vi "SMU.Keithley2600.GetResource.vi"(8 "error in (no error)":errorcluster, 11 "SMU.Keithley2600 in":refnum<class "SMU.Keithley2600.lvclass">) -> (0 "error out":errorcluster, 2 "Resource":T1 {"Channel" items=["Channel A", "Channel B"]}, 3 "SMU.Keithley2600 out":refnum<class "SMU.Keithley2600.lvclass">)   [LabVIEW 2017, in "SMU.Keithley2600.lvclass"]
uses:
  SMU.Keithley2600.lvclass
  Typedefs/Resource--Cluster.ctl
  SMU.Keithley2600.lvclass/SMU.Keithley2600.ctl
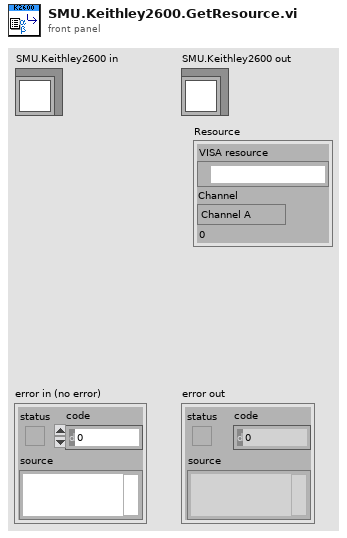
[diagram p1: front panel]
types:
  T1 = typedef "SMU.Keithley2600.lvclass/Resource--Cluster.ctl" = cluster{"VISA resource":refnum<visa-resource-name>, "Channel":i32}
  T2 = typedef "SMU.Keithley2600.lvclass/PrivateData--Ref.ctl" = refnum<data-value>
  T3 = typedef "SMU.Keithley2600.lvclass/PrivateData--Cluster.ctl" = cluster{"Resource":T1}
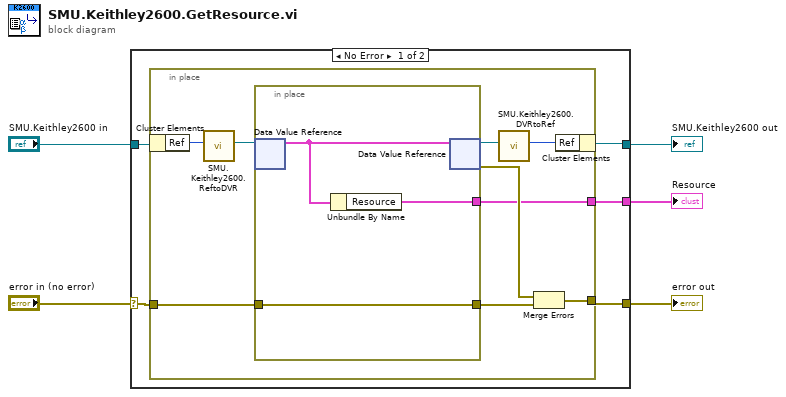
[diagram p0: block diagram]
diagram:
  n1 = case shown="No Error" "error in (no error)" {
    selector: "error in (no error)" -> [w10 w24]
    tunnel: [w9 w24] -> w4
    tunnel: [w8 w23] -> w2
    tunnel: "SMU.Keithley2600 in" -> [w7 w23]
    tunnel: [w6 _] -> w1
    frame No Error {
      n2 = in-place {
        in-place-border: [w16] -> w9
        in-place-border: w10 -> [w14]
        in-place-border: [w11] -> w6
        n3 = in-place-cluster #1(w7) -> ("Ref"=w18:u32)
        n4 = call "SMU.Keithley2600.ReftoDVR.vi"("Ref"=w18) -> ("Ref"=w17:T2)  [unwired: 10 in]
        n5 = in-place {
          in-place-border: w14 -> [w22]
          in-place-border: [w22] -> w13
          in-place-border: [w20] -> w11
          n6 = in-place-dvr #2(w17) -> (w21:T3)  [unwired: 1 out]
          n7 = Unbundle By Name(w21) -> ("Resource"=w20:T1)
          n8 = in-place-dvr #2(w21) -> (w12:T2, w15:errorcluster)
        }
        n9 = call "SMU.Keithley2600.DVRtoRef.vi"("Ref"=w12) -> ("Ref"=w19:u32)  [unwired: 10 in]
        n10 = Merge Errors(w15, w13) -> (w16:errorcluster)
        n11 = in-place-cluster #1("Ref"=w19) -> (w8:refnum<class "SMU.Keithley2600.lvclass">)
      }
    }
    frame Error {
    }
  }
  "error out" <- w4
  "SMU.Keithley2600 out" <- w2
  "Resource" <- w1
